vi "OF state PUSH.vi"(8 "errin":errorcluster, 10 "OF":string, 11 "result":string) -> (0 "error out":errorcluster)   [LabVIEW 2020]
doc: "Incremente l'état de l'OF"
uses:
  <userlib>/Sylvain.lib/DATA_INSERT.vi
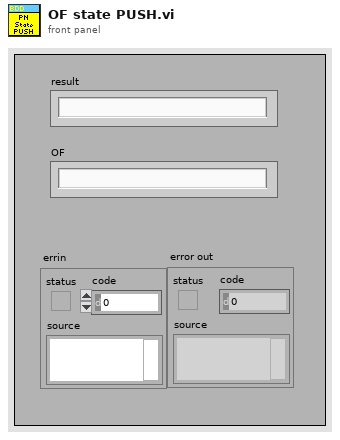
[diagram p1: front panel]
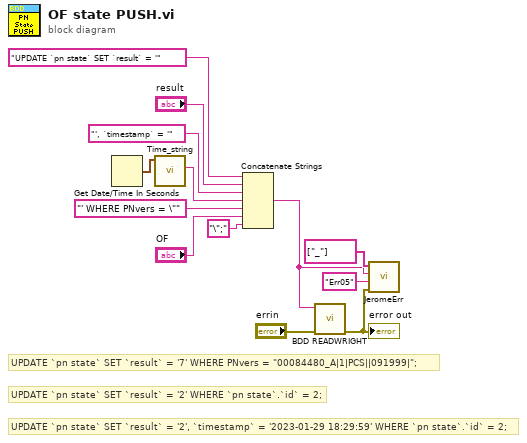
[diagram p0: block diagram]
diagram:
  # "UPDATE `pn state` SET `result` = '2', `timestamp` = '2023-01-29 18:29:59' WHERE `pn state`.`id` = 2;"
  # "UPDATE `pn state` SET `result` = '7' WHERE PNvers = \"00084480_A|1|PCS||091999|\";"
  # "UPDATE `pn state` SET `result` = '2' WHERE `pn state`.`id` = 2;"
  n1 = Get Date/Time In Seconds() -> (seconds since 1Jan1904=w8:timestamp)
  n2 = call <userlib>:"Time_string.vi"("h in"=w8) -> ("heure sql"=w7:string)  [unwired: 9 in, 1 out]
  n3 = Concatenate Strings("UPDATE `pn state` SET `result` = '" ("SQL query"), "result", "', `timestamp` = '" ("chaîne"), w7, "' WHERE PNvers = \"" ("chaîne"), "OF", "\";" ("chaîne")) -> (w1:string)
  n4 = call "BDD READWRIGHT.vi"("errin"="errin", "INSERT"=w1) -> ("errout"=w2:errorcluster)  [unwired: 9 in]
  "error out" <- w2
  n5 = call "JeromeErr.vi"("Errin"=w2, "CodeERR"="Err05", "RequetteSQL"=w1, "RetourSQL"=string[] ["_"]) -> ()  [unwired: 7 in, 1 out]
